vi "Perform Action.vi"(8 "error in":errorcluster, 10 "Input":variant, 11 "Virt Instrument Base in":refnum<class "Virt HSU MCU All Signals Reader.lvclass">) -> (0 "error out":errorcluster, 2 "Output":variant, 3 "Virt Instrument Base out":refnum<class "Virt HSU MCU All Signals Reader.lvclass">)   [LabVIEW 2023, in "Virt HSU MCU All Signals Reader.lvclass"]
uses:
  Virt HSU MCU All Signals Reader.lvclass
  Virt HSU MCU All Signals Reader.lvclass/Virt HSU MCU All Signals Reader.ctl
  Virt Instr Host/Virt Instr Local.lvclass
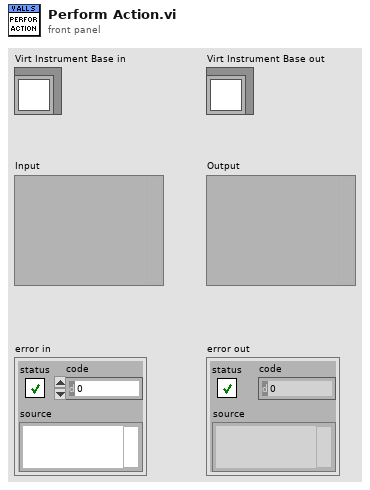
[diagram p1: front panel]
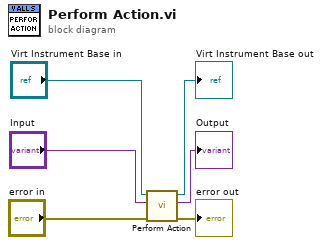
[diagram p0: block diagram]
diagram:
  n1 = call-parent "Perform Action.vi"("error in"="error in", "Input"="Input", "Virt Instrument Base in"="Virt Instrument Base in") -> ("error out"=→"error out":errorcluster, "Output"=→"Output":variant, "Virt Instrument Base out"=→"Virt Instrument Base out":refnum<class "Virt HSU MCU All Signals Reader.lvclass">)  [unwired: 6 in]
